vi "Charge.Wait.Discharge_3P_Repeat.vi"() -> ()   [LabVIEW 2020]
uses:
  <instrlib>/NH Research Regenerative Test Series/Public/Configure/Output Safety.ctl
  <vilib>/DAQmx/read.llb/DAQmx Read (Analog 1D DBL NChan 1Samp).vi
  <vilib>/DAQmx/miscellaneous.llb/DAQmx Fill In Error Info.vi
  <instrlib>/NH Research Regenerative Test Series/Public/Data/Read (Ave Current).vi
  <instrlib>/NH Research Regenerative Test Series/Public/Data/Low Level/Fetch (Ave Voltage).vi
  <instrlib>/NH Research Regenerative Test Series/Public/Data/Low Level/Fetch (Ave True Power).vi
  <instrlib>/NH Research Regenerative Test Series/NH Research Regenerative Test Series.lvlib
panel:
  in  "Starting Cycle":i32
  in  "Discharge Folder Path":path
  in  "Charge Folder Path":path
  out "Cycle Index":i32
  in  "Number Of cycles":dbl
  out "Filename Out 5":path caption="Filename Out"
  out "Ave Current (A) 4":dbl
  out "Ave Voltage (V) 4":dbl
  out "Ave True Power (W) 4":dbl
  out "Status Byte Register 4":T1
  out "WaitElapsed Time (s) 2":dbl caption="Elapsed Time (s)"
  out "Battery3dischargeCurrent":dbl
  out "Battery3chargeCurrent":dbl
  in  "Discharge Voltage Setpoint (0 V)":dbl
  out "Task error out":errorcluster
  out "String":string
  out "Filename Out 3":path caption="Filename Out"
  out "Ave Current (A) 3":dbl
  out "Ave Voltage (V) 3":dbl
  out "Ave True Power (W) 3":dbl
  out "Status Byte Register 3":T1
  out "Current Compare dis":dbl
  out "Battery1dischargeCurrent":dbl
  out "Battery2dischargeCurrent":dbl
  in  "Wait time":dbl
  out "Filename Out 2":path caption="Filename Out"
  out "Ave Current (A) 2":dbl
  out "Ave Voltage (V) 2":dbl
  out "Ave True Power (W) 2":dbl
  out "Status Byte Register 2":T1
  out "WaitElapsed Time (s)":dbl caption="Elapsed Time (s)"
  in  "C rate Setpoint":dbl format="%#.6g"
  in  "Output Safety":T2
  out "Filename Out":path
  in  "DAQmx Task Name":refnum<k21>
  in  "Current Cutoff":dbl
  out "Ave Current (A)":dbl
  out "Ave Voltage (V)":dbl
  out "Ave True Power (W)":dbl
  out "Status Byte Register":T1
  out "Current Compare":dbl
  out "Battery1ChargeCurrent":dbl
  out "Battery2chargeCurrent":dbl
  out "BatteryTempExt":dbl
  in  "Logical Instrument Number":u32=1
  in  "Capacity Setpoint":dbl format="%#.6g"
  in  "Charge Voltage Setpoint":dbl format="%#.6g"
  in  "VISA resource name":refnum<visa-resource-name>
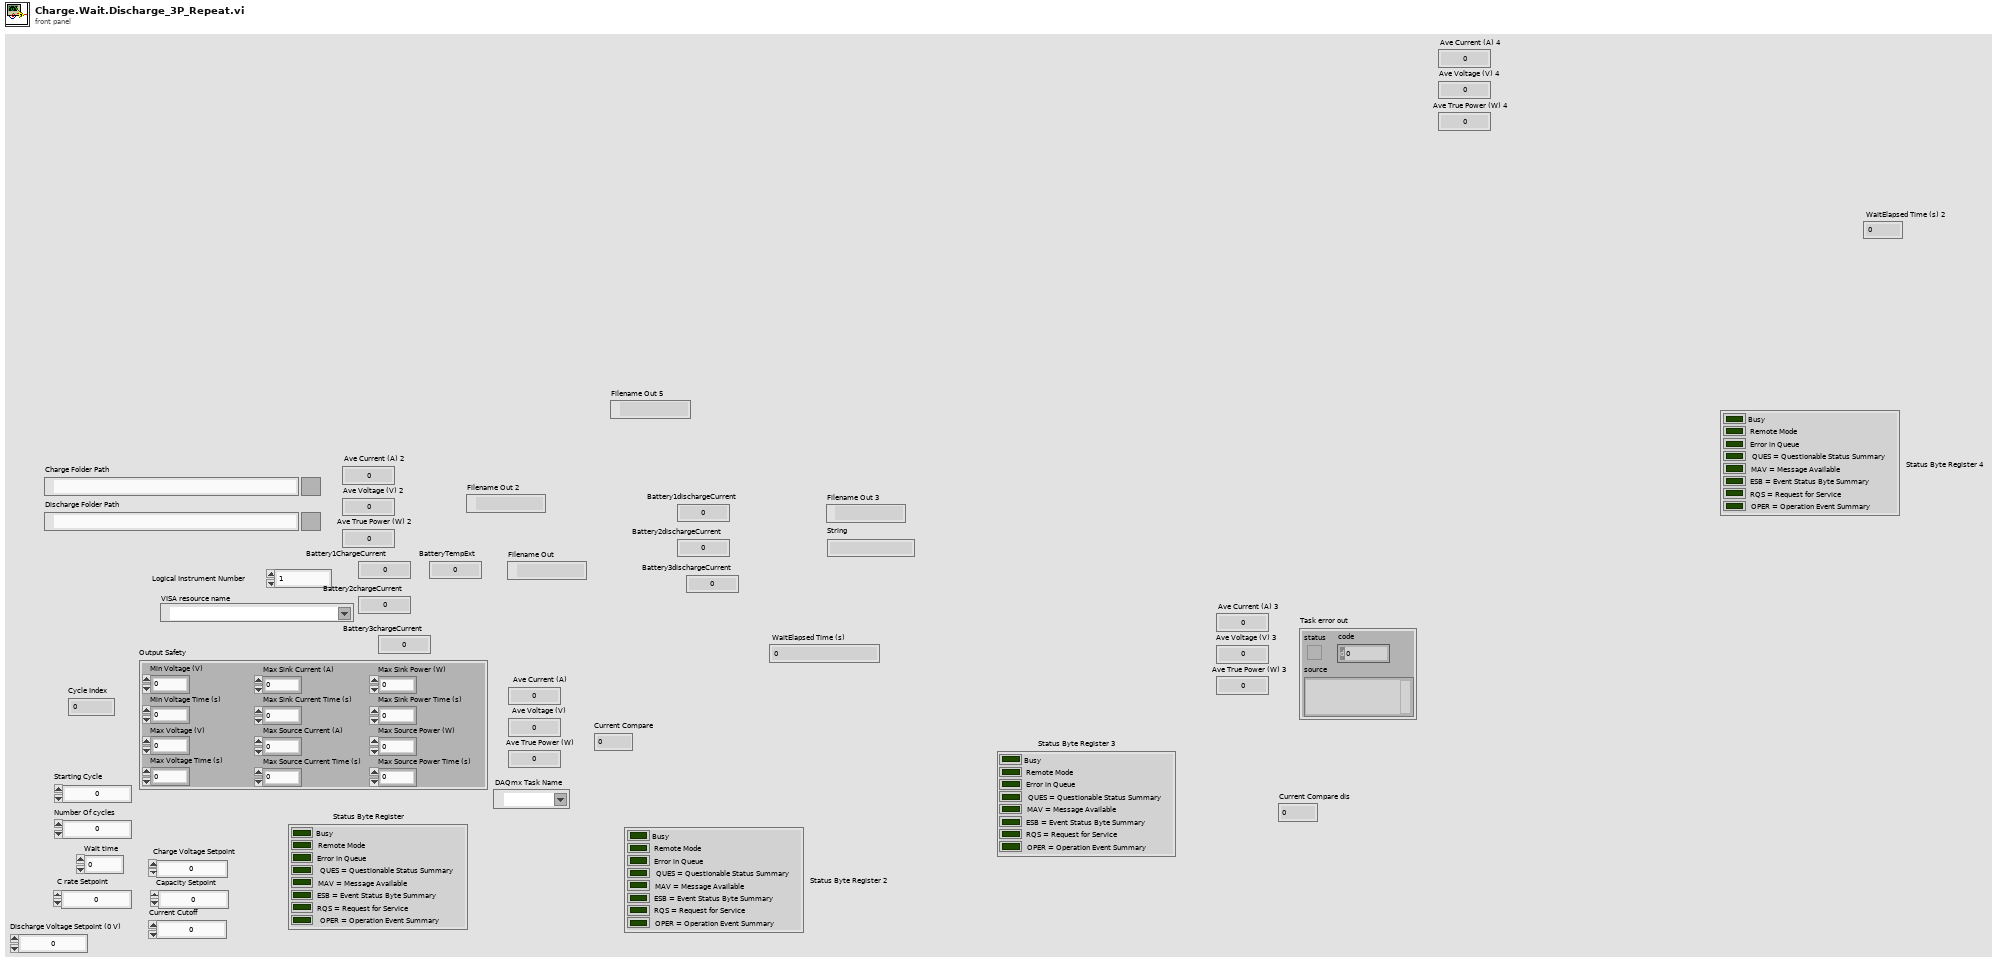
[diagram p1: front panel]
types:
  T1 = cluster{"Busy":bool, "Remote Mode":bool, "Error in Queue":bool, "QUES = Questionable Status Summary":bool, "MAV = Message Available":bool, "ESB = Event Status Byte Summary":bool, "RQS = Request for Service":bool, "OPER = Operation Event Summary":bool}
  T2 = typedef "NH Research Regenerative Test Series.lvlib/Output Safety.ctl" = cluster{"Min Voltage (V)":dbl, "Min Voltage Time (s)":dbl, "Max Voltage (V)":dbl, "Max Voltage Time (s)":dbl, "Max Sink Current (A)":dbl, "Max Sink Current Time (s)":dbl, "Max Source Current (A)":dbl, "Max Source Current Time (s)":dbl, "Max Sink Power (W)":dbl, "Max Sink Power Time (s)":dbl, "Max Source Power (W)":dbl, "Max Source Power Time (s)":dbl}
  T3 = cluster{"data[0]":dbl, "data[1]":dbl, "data[2]":dbl, "data[3]":dbl, "data[4]":dbl, "data[5]":dbl, "data[6]":dbl, "data[7]":dbl, "data[8]":dbl, "data[9]":dbl}
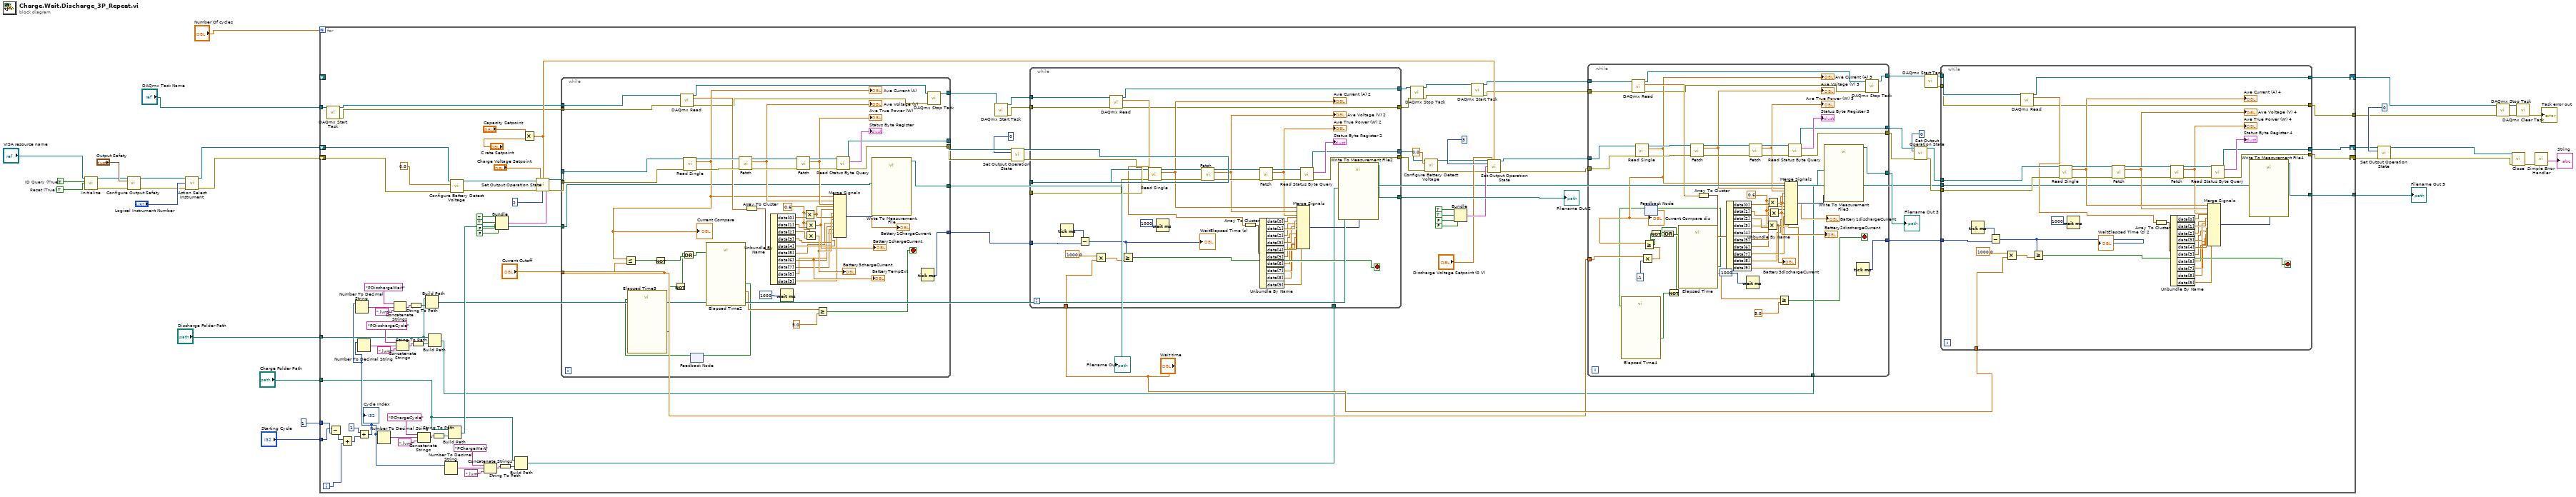
[diagram p0: block diagram]
diagram:
  w4 = TRUE  # ID Query (True)
  w3 = TRUE  # Reset (True)
  n1 = call <vilib>:"Initialize.vi"("VISA resource name"="VISA resource name", "ID Query (True)"=w4, "Reset (True)"=w3) -> ("VISA resource name out"=w1:refnum<visa-resource-name>, "error out"=w2:errorcluster)  [unwired: 11 in]
  n2 = call <instrlib>:"Configure Output Safety.vi"("VISA resource name"=w1, "Output Safety"="Output Safety", "error in (no error)"=w2) -> ("VISA resource name out"=w28:refnum<visa-resource-name>, "error out"=w27:errorcluster)  [unwired: 11 in]
  n3 = call <instrlib>:"Action Select Instrument.vi"("VISA resource name"=w28, "Logical Instrument Number"="Logical Instrument Number", "error in (no error)"=w27) -> ("VISA resource name out"=w10:refnum<visa-resource-name>, "error out"=w9:errorcluster)  [unwired: 11 in]
  n4 = for {
    N: "Number Of cycles" -> [_]
    tunnel: [w98] -> w17
    tunnel: [w95] -> w14
    shift-right: [w97] -> w16
    shift-left: w10 -> [w61]
    shift-right: [w96] -> w15
    shift-left: w9 -> [w60]
    shift-right: [w99] -> w18
    shift-left: _ -> [_]
    tunnel: "Charge Folder Path" -> [w52]
    tunnel: "Discharge Folder Path" -> [w51]
    tunnel: "Starting Cycle" -> [w40]
    tunnel: 1 -> [w41]
    tunnel: "DAQmx Task Name" -> [w37]
    i -> [w42]
    n5 = call <vilib>:"DAQmx Start Task.vi"("task/channels in"=w37) -> ("task out"=w36:refnum<k21>, "error out"=w35:errorcluster)  [unwired: 13 in]
    n6 = Subtract(x=w40, y=w41) -> (x-y=w39:i32)
    n7 = Add(x=w39, y=w42) -> (x+y=w38:i32)
    n8 = Add(x=1, y=w38) -> (x+y=w69:i32)
    "Cycle Index" <- w69
    n9 = Number To Decimal String(number=w69) -> (decimal integer string=w76:string)  [unwired: 1 in]
    n10 = Number To Decimal String(number=w69) -> (decimal integer string=w81:string)  [unwired: 1 in]
    n11 = Number To Decimal String(number=w69) -> (decimal integer string=w86:string)  [unwired: 1 in]
    n12 = Concatenate Strings("PDischargeWait", w76, ".lvm") -> (w77:string)
    n13 = Concatenate Strings("PDischargeCycle", w81, ".lvm") -> (w82:string)
    n14 = String To Path(string=w77) -> (path=w78:path)
    n15 = String To Path(string=w82) -> (path=w83:path)
    n16 = Concatenate Strings("PChargeCycle", w86, ".lvm") -> (w87:string)
    n17 = Build Path(base path=w51, name or relative path=w78) -> (appended path=w53:path)
    n18 = Build Path(base path=w51, name or relative path=w83) -> (appended path=w54:path)
    n19 = String To Path(string=w87) -> (path=w88:path)
    n20 = Number To Decimal String(number=w69) -> (decimal integer string=w71:string)  [unwired: 1 in]
    n21 = Build Path(base path=w52, name or relative path=w88) -> (appended path=w56:path)
    n22 = call <instrlib>:"Configure Battery Detect Voltage.vi"("VISA resource name"=w61, "Battery Detect Voltage (0V)"=0.0, "error in (no error)"=w60) -> ("VISA resource name out"=w59:refnum<visa-resource-name>, "error out"=w58:errorcluster)  [unwired: 11 in]
    n23 = Concatenate Strings("PChargeWait", w71, ".lvm") -> (w72:string)
    n24 = Bundle(TRUE, TRUE, FALSE, FALSE) -> (w120:cluster{bool, bool, bool, bool})  [unwired: 1 in]
    n25 = String To Path(string=w72) -> (path=w73:path)
    n26 = Build Path(base path=w52, name or relative path=w73) -> (appended path=w55:path)
    n27 = Multiply(x="Capacity Setpoint", y="C rate Setpoint") -> (x*y=w105:dbl)
    n28 = call <vilib>:"Set Output Operation State.vi"("VISA resource name"=w59, "Voltage Setpoint (0 V)"="Charge Voltage Setpoint", "Current Setpoint (0 A)"=w105, "Mode (0: Off)"=2, "Enable"=w120, "error in (no error)"=w58) -> ("VISA resource name out"=w127:refnum<visa-resource-name>, "error out"=w126:errorcluster)  [unwired: 8 in]
    n29 = while {
      tunnel: w127 -> [w311]
      tunnel: w126 -> [w310]
      tunnel: [w308] -> w130
      tunnel: [w307] -> w129
      tunnel: "Current Cutoff" -> [w301]
      tunnel: [w302] -> w119
      tunnel: [w282] -> w68
      tunnel: w56 -> [w277]
      tunnel: [w269] -> w44
      tunnel: w36 -> [w268]
      tunnel: w35 -> [w267]
      stop <- w274 stop-if-true
      w291 = 0.6
      n30 = call-poly <vilib>:"DAQmx Read.vi"("task/channels in"=w268, "error in"=w267) -> ("task out"=w271:refnum<k21>, "data"=w305:dbl[], "error out"=w270:errorcluster)  [unwired: 11 in]
      n31 = call-poly <instrlib>:"Read Single.vi"("VISA resource name"=w311, "error in (no error)"=w310) -> ("VISA resource name out"=w316:refnum<visa-resource-name>, "Ave Current (A)"=w299:dbl, "error out"=w317:errorcluster)  [unwired: 11 in]
      "Ave Current (A)" <- w299
      "Current Compare" <- w299
      n32 = Less Or Equal?(x=w299, y=w301) -> (x <= y?=w290:bool)
      n33 = Not(x=w290) -> (.not. x?=w281:bool)
      n34 = feedback #1() -> (w272:bool)  [unwired: 1 in]
      n35 = call "Elapsed Time3"("Reset"=w272) -> ("Time has Elapsed"=w280:bool)  [unwired: 11 in, 7 out]
      n36 = Not(x=w280) -> (.not. x?=w279:bool)
      n37 = Or(x=w279, y=w281) -> (x .or. y?=w278:bool)
      n38 = call "Elapsed Time2"("Reset"=w278) -> ("Elapsed Time (s)"=w276:dbl, "Time has Elapsed"=w273:bool)  [unwired: 11 in, 6 out]
      n39 = feedback-in #1(w273) -> ()
      n40 = call-poly <instrlib>:"Fetch.vi"("VISA resource name"=w316, "error in (no error)"=w317) -> ("VISA resource name out"=w315:refnum<visa-resource-name>, "Ave Voltage (V)"=w300:dbl, "error out"=w314:errorcluster)  [unwired: 11 in]
      "Ave Voltage (V)" <- w300
      n41 = Array To Cluster(array=w305) -> (cluster=w304:T3)
      n42 = Unbundle By Name(w304) -> ("data[0]"=w297:dbl, "data[1]"=w295:dbl, "data[2]"=w292:dbl, "data[3]"=w289:dbl, "data[4]"=w288:dbl, "data[5]"=w287:dbl, "data[6]"=w286:dbl, "data[7]"=w285:dbl, "data[8]"=w284:dbl, "data[9]"=w283:dbl)
      "BatteryTempExt" <- w286
      n43 = Wait (ms)(milliseconds to wait=1000) -> ()  [unwired: 1 out]
      n44 = call-poly <instrlib>:"Fetch.vi"("VISA resource name"=w315, "error in (no error)"=w314) -> ("VISA resource name out"=w313:refnum<visa-resource-name>, "Ave True Power (W)"=w306:dbl, "error out"=w312:errorcluster)  [unwired: 11 in]
      "Ave True Power (W)" <- w306
      n45 = Multiply(x=w291, y=w297) -> (x*y=w296:dbl)
      "Battery1ChargeCurrent" <- w296
      n46 = Multiply(x=w291, y=w295) -> (x*y=w294:dbl)
      "Battery2chargeCurrent" <- w294
      n47 = Multiply(x=w291, y=w292) -> (x*y=w293:dbl)
      "Battery3chargeCurrent" <- w293
      n48 = Greater Or Equal?(x=w276, y=5.0) -> (x >= y?=w274:bool)
      n49 = Merge Signals "Merge Signals"(w299, w300, w306, w296, w294, w293, w289, w288, w287, w286, w285, w284, w283) -> (w303:dynamicdata)
      n50 = call <instrlib>:"Read Status Byte Query.vi"("VISA resource name"=w313, "error in (no error)"=w312) -> ("VISA resource name out"=w308:refnum<visa-resource-name>, "Status Byte Register"=→"Status Byte Register":T1, "error out"=w307:errorcluster)  [unwired: 11 in]
      n51 = call "Write To Measurement File"("Signals"=w303, "Filename"=w277) -> ("Filename Out"=w302:path)  [unwired: 15 in, 2 out]
      n52 = Tick Count (ms)() -> (millisecond timer value=w282:u32)
      n53 = call <vilib>:"DAQmx Stop Task.vi"("task/channels in"=w271, "error in"=w270) -> ("task out"=w269:refnum<k21>)  [unwired: 12 in, 1 out]
    }
    "Filename Out" <- w119
    n54 = call <vilib>:"DAQmx Start Task.vi"("task/channels in"=w44) -> ("task out"=w50:refnum<k21>, "error out"=w49:errorcluster)  [unwired: 13 in]
    n55 = call <vilib>:"Set Output Operation State.vi"("VISA resource name"=w130, "Mode (0: Off)"=0, "error in (no error)"=w129) -> ("VISA resource name out"=w116:refnum<visa-resource-name>, "error out"=w115:errorcluster)  [unwired: 11 in]
    n56 = while {
      tunnel: w116 -> [w259]
      tunnel: w115 -> [w258]
      tunnel: [w256] -> w63
      tunnel: [w255] -> w64
      tunnel: "Wait time" -> [w242]
      tunnel: w68 -> [w244]
      tunnel: [w239] -> w117
      tunnel: w55 -> [w230]
      tunnel: w50 -> [w229]
      tunnel: w49 -> [w228]
      tunnel: [w227] -> w34
      tunnel: [w226] -> w33
      stop <- w245 stop-if-true
      n57 = Tick Count (ms)() -> (millisecond timer value=w246:u32)
      n58 = Subtract(x=w246, y=w244) -> (x-y=w243:u32)
      "WaitElapsed Time (s)" <- w243
      n59 = Multiply(x=1000.0, y=w242) -> (x*y=w240:dbl)
      n60 = call-poly <vilib>:"DAQmx Read.vi"("task/channels in"=w229, "error in"=w228) -> ("task out"=w227:refnum<k21>, "data"=w251:dbl[], "error out"=w226:errorcluster)  [unwired: 11 in]
      n61 = Greater Or Equal?(x=w243, y=w240) -> (x >= y?=w245:bool)
      n62 = call-poly <instrlib>:"Read Single.vi"("VISA resource name"=w259, "error in (no error)"=w258) -> ("VISA resource name out"=w264:refnum<visa-resource-name>, "Ave Current (A)"=w254:dbl, "error out"=w265:errorcluster)  [unwired: 11 in]
      "Ave Current (A) 2" <- w254
      n63 = Wait (ms)(milliseconds to wait=1000) -> ()  [unwired: 1 out]
      n64 = call-poly <instrlib>:"Fetch.vi"("VISA resource name"=w264, "error in (no error)"=w265) -> ("VISA resource name out"=w263:refnum<visa-resource-name>, "Ave Voltage (V)"=w253:dbl, "error out"=w262:errorcluster)  [unwired: 11 in]
      "Ave Voltage (V) 2" <- w253
      n65 = Array To Cluster(array=w251) -> (cluster=w250:T3)
      n66 = call-poly <instrlib>:"Fetch.vi"("VISA resource name"=w263, "error in (no error)"=w262) -> ("VISA resource name out"=w261:refnum<visa-resource-name>, "Ave True Power (W)"=w252:dbl, "error out"=w260:errorcluster)  [unwired: 11 in]
      "Ave True Power (W) 2" <- w252
      n67 = Unbundle By Name(w250) -> ("data[0]"=w249:dbl, "data[1]"=w248:dbl, "data[2]"=w238:dbl, "data[3]"=w237:dbl, "data[4]"=w236:dbl, "data[5]"=w235:dbl, "data[6]"=w234:dbl, "data[7]"=w233:dbl, "data[8]"=w232:dbl, "data[9]"=w231:dbl)
      n68 = Merge Signals "Merge Signals"(w254, w253, w252, w249, w248, w238, w237, w236, w235, w234, w233, w232, w231) -> (w266:dynamicdata)
      n69 = call <instrlib>:"Read Status Byte Query.vi"("VISA resource name"=w261, "error in (no error)"=w260) -> ("VISA resource name out"=w256:refnum<visa-resource-name>, "Status Byte Register"=→"Status Byte Register 2":T1, "error out"=w255:errorcluster)  [unwired: 11 in]
      n70 = call "Write To Measurement File2"("Signals"=w266, "Filename"=w230) -> ("Filename Out"=w239:path)  [unwired: 15 in, 2 out]
    }
    "Filename Out 2" <- w117
    n71 = call <vilib>:"DAQmx Stop Task.vi"("task/channels in"=w34, "error in"=w33) -> ("task out"=w32:refnum<k21>, "error out"=w31:errorcluster)  [unwired: 12 in]
    n72 = call <instrlib>:"Configure Battery Detect Voltage.vi"("VISA resource name"=w63, "Battery Detect Voltage (0V)"=0.0, "error in (no error)"=w64) -> ("VISA resource name out"=w66:refnum<visa-resource-name>, "error out"=w65:errorcluster)  [unwired: 11 in]
    n73 = Bundle(TRUE, TRUE, FALSE, FALSE) -> (w108:cluster{bool, bool, bool, bool})  [unwired: 1 in]
    n74 = call <vilib>:"DAQmx Start Task.vi"("task/channels in"=w32, "error in"=w31) -> ("task out"=w48:refnum<k21>, "error out"=w47:errorcluster)  [unwired: 12 in]
    n75 = call <vilib>:"Set Output Operation State.vi"("VISA resource name"=w66, "Voltage Setpoint (0 V)"="Discharge Voltage Setpoint (0 V)", "Current Setpoint (0 A)"=w105, "Mode (0: Off)"=3, "Enable"=w108, "error in (no error)"=w65) -> ("VISA resource name out"=w113:refnum<visa-resource-name>, "error out"=w114:errorcluster)  [unwired: 8 in]
    n76 = while {
      tunnel: w113 -> [w219]
      tunnel: w114 -> [w218]
      tunnel: [w216] -> w104
      tunnel: [w215] -> w103
      tunnel: "Current Cutoff" -> [w198]
      tunnel: [w210] -> w94
      tunnel: [w188] -> w57
      tunnel: w54 -> [w187]
      tunnel: w48 -> [w177]
      tunnel: w47 -> [w176]
      tunnel: [w173] -> w43
      stop <- w180 stop-if-true
      w203 = 0.6
      n77 = call-poly <vilib>:"DAQmx Read.vi"("task/channels in"=w177, "error in"=w176) -> ("task out"=w175:refnum<k21>, "data"=w213:dbl[], "error out"=w174:errorcluster)  [unwired: 11 in]
      n78 = call-poly <instrlib>:"Read Single.vi"("VISA resource name"=w219, "error in (no error)"=w218) -> ("VISA resource name out"=w224:refnum<visa-resource-name>, "Ave Current (A)"=w200:dbl, "error out"=w225:errorcluster)  [unwired: 11 in]
      "Ave Current (A) 3" <- w200
      "Current Compare dis" <- w200
      n79 = Multiply(x=w198, y=-1) -> (x*y=w197:dbl)
      n80 = Greater Or Equal?(x=w200, y=w197) -> (x >= y?=w196:bool)
      n81 = feedback #2() -> (w178:bool)  [unwired: 1 in]
      n82 = call "Elapsed Time4"("Reset"=w178) -> ("Time has Elapsed"=w186:bool)  [unwired: 11 in, 7 out]
      n83 = Not(x=w196) -> (.not. x?=w182:bool)
      n84 = Not(x=w186) -> (.not. x?=w181:bool)
      n85 = Or(x=w181, y=w182) -> (x .or. y?=w183:bool)
      n86 = call "Elapsed Time"("Reset"=w183) -> ("Elapsed Time (s)"=w184:dbl, "Time has Elapsed"=w179:bool)  [unwired: 11 in, 6 out]
      n87 = feedback-in #2(w179) -> ()
      n88 = call-poly <instrlib>:"Fetch.vi"("VISA resource name"=w224, "error in (no error)"=w225) -> ("VISA resource name out"=w223:refnum<visa-resource-name>, "Ave Voltage (V)"=w209:dbl, "error out"=w222:errorcluster)  [unwired: 11 in]
      "Ave Voltage (V) 3" <- w209
      n89 = Array To Cluster(array=w213) -> (cluster=w212:T3)
      n90 = Unbundle By Name(w212) -> ("data[0]"=w207:dbl, "data[1]"=w206:dbl, "data[2]"=w202:dbl, "data[3]"=w195:dbl, "data[4]"=w194:dbl, "data[5]"=w193:dbl, "data[6]"=w192:dbl, "data[7]"=w191:dbl, "data[8]"=w190:dbl, "data[9]"=w189:dbl)
      n91 = Wait (ms)(milliseconds to wait=1000) -> ()  [unwired: 1 out]
      n92 = call-poly <instrlib>:"Fetch.vi"("VISA resource name"=w223, "error in (no error)"=w222) -> ("VISA resource name out"=w221:refnum<visa-resource-name>, "Ave True Power (W)"=w214:dbl, "error out"=w220:errorcluster)  [unwired: 11 in]
      "Ave True Power (W) 3" <- w214
      n93 = Multiply(x=w203, y=w202) -> (x*y=w201:dbl)
      "Battery3dischargeCurrent" <- w201
      n94 = Multiply(x=w203, y=w207) -> (x*y=w205:dbl)
      "Battery1dischargeCurrent" <- w205
      n95 = Multiply(x=w203, y=w206) -> (x*y=w204:dbl)
      "Battery2dischargeCurrent" <- w204
      n96 = Greater Or Equal?(x=w184, y=5.0) -> (x >= y?=w180:bool)
      n97 = Merge Signals "Merge Signals"(w200, w209, w214, w205, w204, w201, w195, w194, w193, w192, w191, w190, w189) -> (w211:dynamicdata)
      n98 = call <instrlib>:"Read Status Byte Query.vi"("VISA resource name"=w221, "error in (no error)"=w220) -> ("VISA resource name out"=w216:refnum<visa-resource-name>, "Status Byte Register"=→"Status Byte Register 3":T1, "error out"=w215:errorcluster)  [unwired: 11 in]
      n99 = call "Write To Measurement File3"("Signals"=w211, "Filename"=w187) -> ("Filename Out"=w210:path)  [unwired: 15 in, 2 out]
      n100 = Tick Count (ms)() -> (millisecond timer value=w188:u32)
      n101 = call <vilib>:"DAQmx Stop Task.vi"("task/channels in"=w175, "error in"=w174) -> ("task out"=w173:refnum<k21>)  [unwired: 12 in, 1 out]
    }
    "Filename Out 3" <- w94
    n102 = call <vilib>:"Set Output Operation State.vi"("VISA resource name"=w104, "Mode (0: Off)"=0, "error in (no error)"=w103) -> ("VISA resource name out"=w101:refnum<visa-resource-name>, "error out"=w100:errorcluster)  [unwired: 11 in]
    n103 = call <vilib>:"DAQmx Start Task.vi"("task/channels in"=w43) -> ("task out"=w46:refnum<k21>, "error out"=w45:errorcluster)  [unwired: 13 in]
    n104 = while {
      tunnel: w101 -> [w165]
      tunnel: w100 -> [w164]
      tunnel: [w162] -> w97
      tunnel: [w161] -> w96
      tunnel: "Wait time" -> [w148]
      tunnel: w57 -> [w150]
      tunnel: [w145] -> w98
      tunnel: [w144] -> w99
      tunnel: [w143] -> w95
      tunnel: w53 -> [w134]
      tunnel: w46 -> [w133]
      tunnel: w45 -> [w132]
      stop <- w151 stop-if-true
      n105 = Tick Count (ms)() -> (millisecond timer value=w152:u32)
      n106 = Subtract(x=w152, y=w150) -> (x-y=w149:u32)
      "WaitElapsed Time (s) 2" <- w149
      n107 = Multiply(x=1000.0, y=w148) -> (x*y=w146:dbl)
      n108 = call-poly <vilib>:"DAQmx Read.vi"("task/channels in"=w133, "error in"=w132) -> ("task out"=w144:refnum<k21>, "data"=w157:dbl[], "error out"=w145:errorcluster)  [unwired: 11 in]
      n109 = Greater Or Equal?(x=w149, y=w146) -> (x >= y?=w151:bool)
      n110 = call-poly <instrlib>:"Read Single.vi"("VISA resource name"=w165, "error in (no error)"=w164) -> ("VISA resource name out"=w170:refnum<visa-resource-name>, "Ave Current (A)"=w160:dbl, "error out"=w171:errorcluster)  [unwired: 11 in]
      "Ave Current (A) 4" <- w160
      n111 = Wait (ms)(milliseconds to wait=1000) -> ()  [unwired: 1 out]
      n112 = call-poly <instrlib>:"Fetch.vi"("VISA resource name"=w170, "error in (no error)"=w171) -> ("VISA resource name out"=w169:refnum<visa-resource-name>, "Ave Voltage (V)"=w159:dbl, "error out"=w168:errorcluster)  [unwired: 11 in]
      "Ave Voltage (V) 4" <- w159
      n113 = Array To Cluster(array=w157) -> (cluster=w156:T3)
      n114 = call-poly <instrlib>:"Fetch.vi"("VISA resource name"=w169, "error in (no error)"=w168) -> ("VISA resource name out"=w167:refnum<visa-resource-name>, "Ave True Power (W)"=w158:dbl, "error out"=w166:errorcluster)  [unwired: 11 in]
      "Ave True Power (W) 4" <- w158
      n115 = Unbundle By Name(w156) -> ("data[0]"=w155:dbl, "data[1]"=w154:dbl, "data[2]"=w142:dbl, "data[3]"=w141:dbl, "data[4]"=w140:dbl, "data[5]"=w139:dbl, "data[6]"=w138:dbl, "data[7]"=w137:dbl, "data[8]"=w136:dbl, "data[9]"=w135:dbl)
      n116 = Merge Signals "Merge Signals"(w160, w159, w158, w155, w154, w142, w141, w140, w139, w138, w137, w136, w135) -> (w172:dynamicdata)
      n117 = call <instrlib>:"Read Status Byte Query.vi"("VISA resource name"=w167, "error in (no error)"=w166) -> ("VISA resource name out"=w162:refnum<visa-resource-name>, "Status Byte Register"=→"Status Byte Register 4":T1, "error out"=w161:errorcluster)  [unwired: 11 in]
      n118 = call "Write To Measurement File4"("Signals"=w172, "Filename"=w134) -> ("Filename Out"=w143:path)  [unwired: 15 in, 2 out]
    }
  }
  "Filename Out 5" <- w14
  n119 = call <vilib>:"Set Output Operation State.vi"("VISA resource name"=w16, "Mode (0: Off)"=0, "error in (no error)"=w15) -> ("VISA resource name out"=w20:refnum<visa-resource-name>, "error out"=w19:errorcluster)  [unwired: 11 in]
  n120 = call <vilib>:"DAQmx Stop Task.vi"("task/channels in"=w18, "error in"=w17) -> ("task out"=w24:refnum<k21>, "error out"=w23:errorcluster)  [unwired: 12 in]
  n121 = call <instrlib>:"Close.vi"("VISA resource name"=w20, "error in (no error)"=w19) -> ("error out"=w21:errorcluster)  [unwired: 13 in]
  n122 = call <vilib>:"DAQmx Clear Task.vi"("task in"=w24, "error in"=w23) -> ("error out"=→"Task error out":errorcluster)  [unwired: 13 in]
  n123 = call <vilib>:"Simple Error Handler.vi"("error in (no error)"=w21) -> ("source out"=→"String":string)  [unwired: 4 in, 4 out]
